vi "Read Pref Value.vi"(8 "error in (no error)":errorcluster, 10 "Pref Hierarchy":string[](array[string]), 11 "Pref Group in":refnum<class "Pref Group.lvclass">) -> (0 "error out":errorcluster, 2 "Value":string, 3 "Pref Group out":refnum<class "Pref Group.lvclass">)   [LabVIEW 2020, in "User Prefs.lvlib" / "Pref Group.lvclass"]
uses:
  Pref Group.lvclass
  Pref Group.lvclass/Pref Group.ctl
  lv-cdm/CDM-Config/Config Manager/Config Manager.lvclass
  lv-cdm/CDM-Config/Config Element/Config Element.lvclass
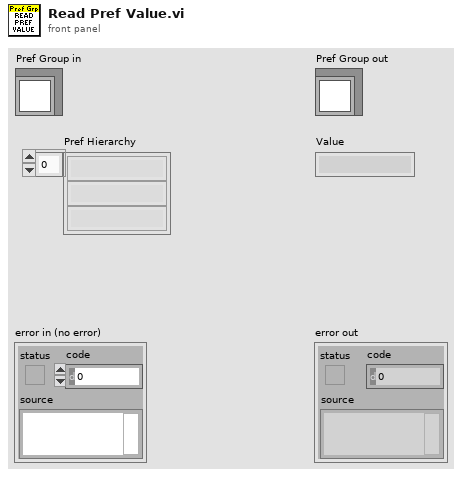
[diagram p1: front panel]
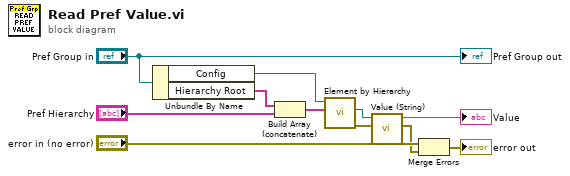
[diagram p0: block diagram]
diagram:
  n1 = Unbundle By Name("Pref Group in") -> ("Config"=w9:refnum<class "Config Manager.lvclass">, "Hierarchy Root"=w1:string[])
  n2 = Build Array (concatenate)(w1, "Pref Hierarchy") -> (w2:string[])
  n3 = call "Element by Hierarchy.vi"("Hierarchy"=w2, "Config Manager in"=w9) -> ("error out"=w6:errorcluster, "Config Element"=w7:refnum<class "Config Element.lvclass">)  [unwired: 7 in, 1 out]
  n4 = call "Value (String).vi"("error in (no error)"=w6, "Config Element in"=w7) -> ("error out"=w3:errorcluster, "String Value"=→"Value":string)  [unwired: 8 in]
  n5 = Merge Errors("error in (no error)", w3) -> (→"error out":errorcluster)
  "Pref Group out" <- "Pref Group in"
